vi "ESPEC config.vi"(8 "error in (no error)":errorcluster, 11 "Parameter":string[](array[string])) -> (0 "error out":errorcluster, 3 "ESPEC":T1={"Ref"=variant, "Configure Parameter"={"Temp Parameter"={"Temperature setpoint"=40.0, "upper limit"=80.0, "lower limit"=0.0}, "Humidity Parameter"={"Humidity setpoint"=50.0, "upper limit"=80.0, "lower limit"=0.0}}})   [LabVIEW 2021, in "Environment Chamber.lvlib"]
uses:
  Environment Chamber.lvlib
  ESPEC Config Parameter.ctl
  Configure Parameter.ctl
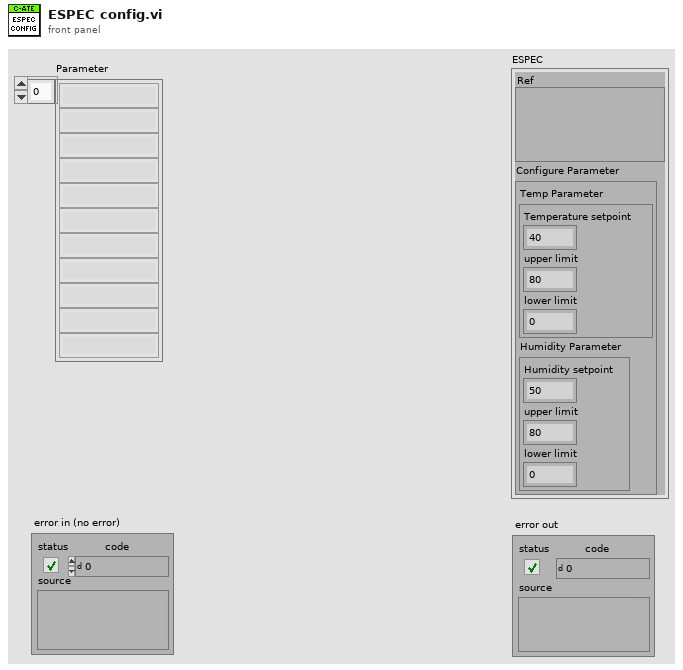
[diagram p1: front panel]
types:
  T1 = typedef "Environment Chamber.lvlib/ESPEC Config Parameter.ctl" = cluster{"Ref":variant, "Configure Parameter":T2}
  T2 = typedef "Environment Chamber.lvlib/Configure Parameter.ctl" = cluster{"Temp Parameter":cluster{"Temperature setpoint":dbl, "upper limit":dbl, "lower limit":dbl}, "Humidity Parameter":cluster{"Humidity setpoint":dbl, "upper limit":dbl, "lower limit":dbl}}
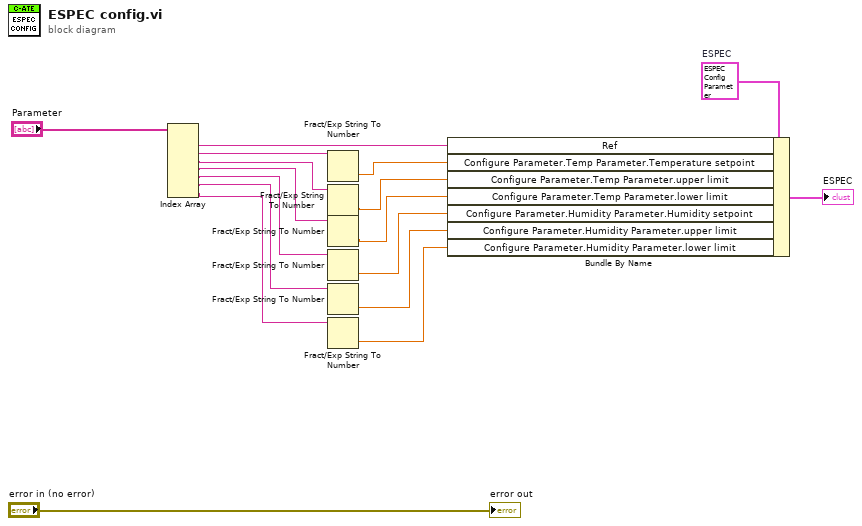
[diagram p0: block diagram]
diagram:
  w16 = T1 {"Ref"=variant, "Configure Parameter"={"Temp Parameter"={"Temperature setpoint"=40.0, "upper limit"=80.0, "lower limit"=0.0}, "Humidity Parameter"={"Humidity setpoint"=50.0, "upper limit"=80.0, "lower limit"=0.0}}}  # ESPEC
  n1 = Index Array(array="Parameter") -> (element #1=w14:string, element #2=w13:string, element #3=w12:string, element #4=w11:string, element #5=w10:string, element #6=w9:string, element #7=w8:string)  [unwired: 7 in]
  n2 = Fract/Exp String To Number(string=w13) -> (number=w7:dbl)  [unwired: 3 in, 1 out]
  n3 = Fract/Exp String To Number(string=w12) -> (number=w6:dbl)  [unwired: 3 in, 1 out]
  n4 = Fract/Exp String To Number(string=w11) -> (number=w5:dbl)  [unwired: 3 in, 1 out]
  n5 = Fract/Exp String To Number(string=w10) -> (number=w4:dbl)  [unwired: 3 in, 1 out]
  n6 = Fract/Exp String To Number(string=w9) -> (number=w3:dbl)  [unwired: 3 in, 1 out]
  n7 = Fract/Exp String To Number(string=w8) -> (number=w2:dbl)  [unwired: 3 in, 1 out]
  n8 = Bundle By Name(cluster=w16, "Ref"=w14, "Configure Parameter.Temp Parameter.Temperature setpoint"=w7, "Configure Parameter.Temp Parameter.upper limit"=w6, "Configure Parameter.Temp Parameter.lower limit"=w5, "Configure Parameter.Humidity Parameter.Humidity setpoint"=w4, "Configure Parameter.Humidity Parameter.upper limit"=w3, "Configure Parameter.Humidity Parameter.lower limit"=w2) -> (→"ESPEC":T1)
  "error out" <- "error in (no error)"
